vi "3_TDMS_View.vi"   [LabVIEW 2014]
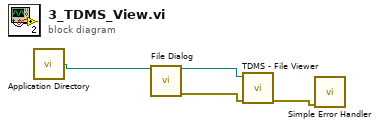
[diagram p0: block diagram]
diagram:
  n1 = call <vilib>:"Application Directory.vi"() -> ("Application Directory"=w4:path)
  n2 = call "File Dialog"("start path"=w4) -> ("selected path"=w3:path, "error out"=w2:errorcluster)  [unwired: 11 in, 2 out]
  n3 = call <vilib>:"TDMS - File Viewer.vi"("error in (no error)"=w2, "file path"=w3) -> ("error out"=w1:errorcluster)  [unwired: 4 in, 1 out]
  n4 = call <vilib>:"Simple Error Handler.vi"("error in (no error)"=w1) -> ()  [unwired: 4 in, 5 out]
